vi "Template Get by Query.vi"(8 "error in (no error)":errorcluster, 10 "Template Query (\"\")":string, 11 "Connection Refnum":T2) -> (0 "error out":errorcluster, 2 "Records":T1[](array[typedef]), 3 "Connection Refnum":T2)   [LabVIEW 2011]
uses:
  Summitek EXT/ODBC/SQL Controls/Connection Refnum.ctl
  Template Record.ctl
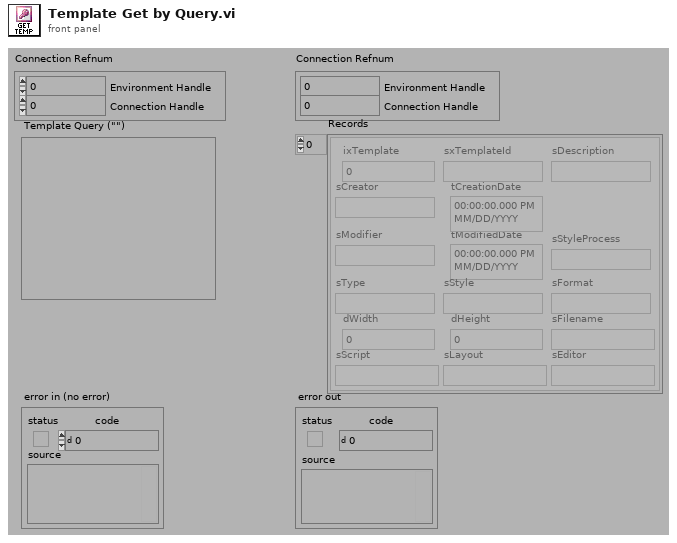
[diagram p1: front panel]
types:
  T1 = typedef "Template Record.ctl" = cluster{"ixTemplate":i32, "sxTemplateId":string, "sDescription":string, "sCreator":string, "tCreationDate":timestamp, "sModifier":string, "tModifiedDate":timestamp, "sType":string, "sStyle":string, "sFormat":string, "dWidth":dbl, "dHeight":dbl, "sFilename":string, "sScript":string, "sLayout":string, "sEditor":string, "sStyleProcess":string}
  T2 = typedef "Connection Refnum.ctl" = cluster{"Environment Handle":i32, "Connection Handle":i32}
  T3 = typedef "Statement Refnum.ctl" = cluster{"Statement Handle":i32, "Parameter Number":u16}
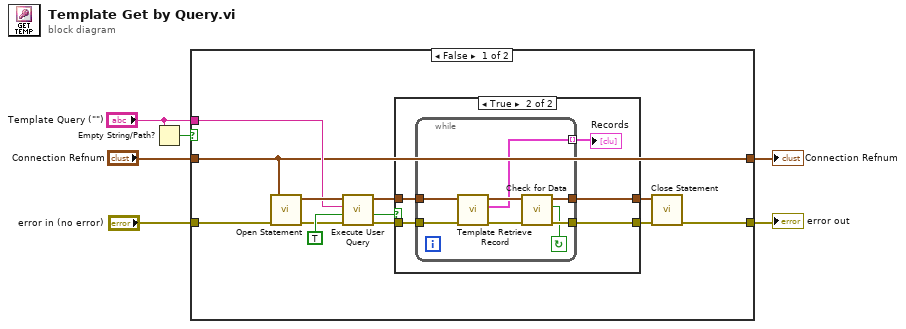
[diagram p0: block diagram]
diagram:
  n1 = Empty String/Path?(string/path="Template Query (\"\")") -> (empty?=w1:bool)
  n2 = case shown="False" w1 {
    tunnel: "error in (no error)" -> [w8 w34]
    tunnel: "Connection Refnum" -> [w7 w35]
    tunnel: [w7 w35] -> w4
    tunnel: [w9 w34] -> w3
    tunnel: "Template Query (\"\")" -> [w10 _]
    frame False {
      n3 = call "Open Statement.vi"("error in (no error)"=w8, "Connection Refnum"=w7) -> ("error out"=w12:errorcluster, "Statement Refnum"=w13:T3)  [unwired: 4 out]
      n4 = call "Execute User Query.vi"("error in (no error)"=w12, "Return Data? (f)"=TRUE, "User Query"=w10, "Statement Refnum"=w13) -> ("error out"=w18:errorcluster, "Data Present?"=w11:bool, "Statement Refnum"=w17:T3)  [unwired: 1 out]
      n5 = case shown="True" w11 {
        tunnel: w18 -> [w19 w24]
        tunnel: w17 -> [w20 w25]
        tunnel: [w19 w22] -> w14
        tunnel: [w20 w23] -> w15
        frame False {
        }
        frame True {
          n6 = while {
            tunnel: w25 -> [w33]
            tunnel: w24 -> [w32]
            tunnel: [w30] -> w23
            tunnel: [w28] -> w22
            tunnel: [w27] -> w21 mode=indexing
            stop <- w26 continue-if-true
            n7 = call "Template Retrieve Record.vi"("error in (no error)"=w32, "Statement Refnum"=w33) -> ("error out"=w29:errorcluster, "Template Record"=w27:T1, "Statement Refnum"=w31:T3)  [unwired: 7 out]
            n8 = call "Check for Data.vi"("error in (no error)"=w29, "Statement Refnum"=w31) -> ("error out"=w28:errorcluster, "Data Present?"=w26:bool, "Statement Refnum"=w30:T3)  [unwired: 3 out]
          }
          "Records" <- w21
        }
      }
      n9 = call "Close Statement.vi"("error in (no error)"=w14, "Statement Refnum"=w15) -> ("error out"=w9:errorcluster)  [unwired: 5 out]
    }
    frame True {
    }
  }
  "error out" <- w3
  "Connection Refnum" <- w4
